vi "IdentifyBlob_Square_Image.vi"(1 "color":u32(colorbox)=16773418, 2 "Centroid":cluster{"X":dbl, "Y":dbl}, 3 "Dimension":i32=20, 4 "picture":picture) -> (0 "picture":picture)   [LabVIEW 2024]
doc: "This VI is used with the BlobTracking.vi or the BiggestComplexBlob.vi. It will draw a shape centered on the blob's centroid. The shape depends upon the shape chosen by the poly selector and the dimension wired to the VI."
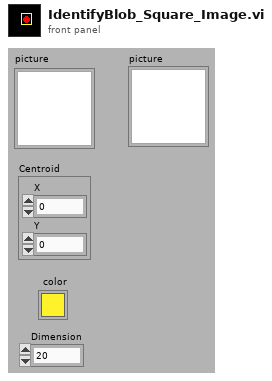
[diagram p1: front panel]
types:
  T1 = cluster{"left":i16, "top":i16, "right":i16, "bottom":i16}
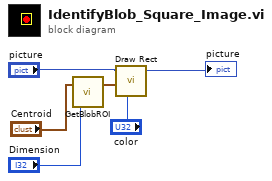
[diagram p0: block diagram]
diagram:
  n1 = call <userlib>:"GetBlobROI.vi"("Dimension"="Dimension", "Centroid"="Centroid") -> ("ROI"=w2:T1)  [unwired: 1 out]
  n2 = call <vilib>:"Draw Rect.vi"("picture"="picture", "rect"=w2, "color(black)"="color") -> ("new picture"=→"picture":picture)  [unwired: 6 in]
